vi "Motion Profile Generator-Target Speed-Demo.vi"(8 "Motion Profile Control Frame Rate":dbl=10.0, 9 "Target Speed":dbl=4.0, 10 "Max Jerk (rotations/sec^2)":dbl=1.0, 11 "Max Acceleration (rotations/sec)":dbl=3.0) -> (0 "XY Graph":cluster{dbl[], dbl[]}[](graph), 1 "jerk rotations/sec^3":dbl[](array[numeric]), 2 "acceleration rotations/sec^2":dbl[](array[numeric]), 3 "velocity rotations/sec":dbl[](array[numeric]))   [LabVIEW 2015]
panel:
  out "Final Speed":dbl
  # "This is just a trapezoidal motion profile generator"
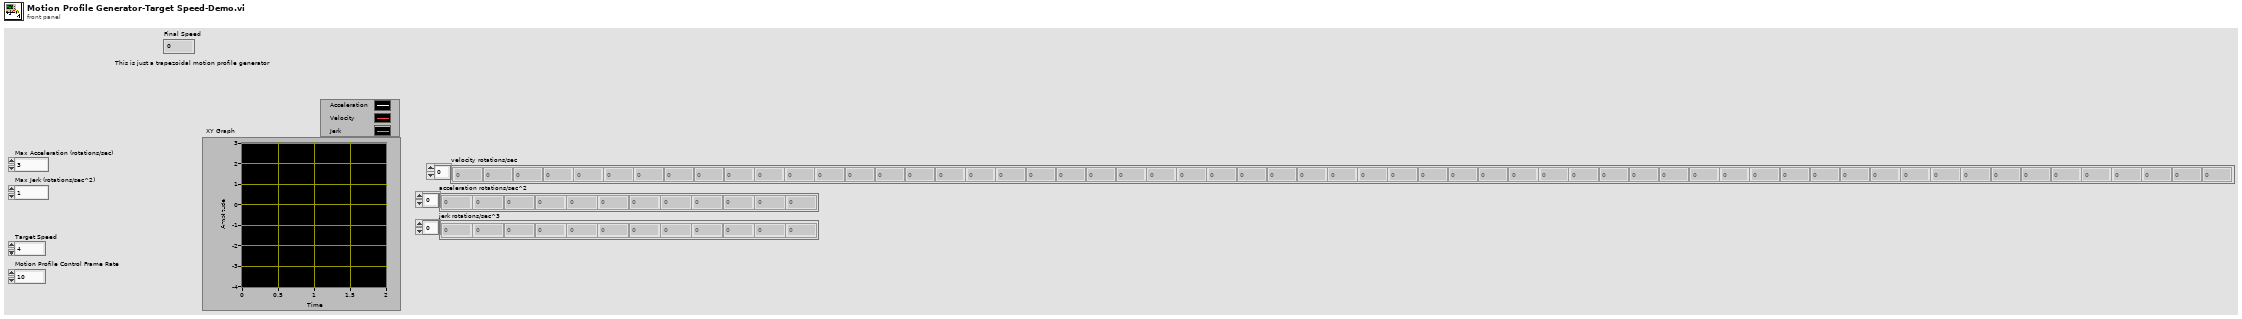
[diagram p1: front panel]
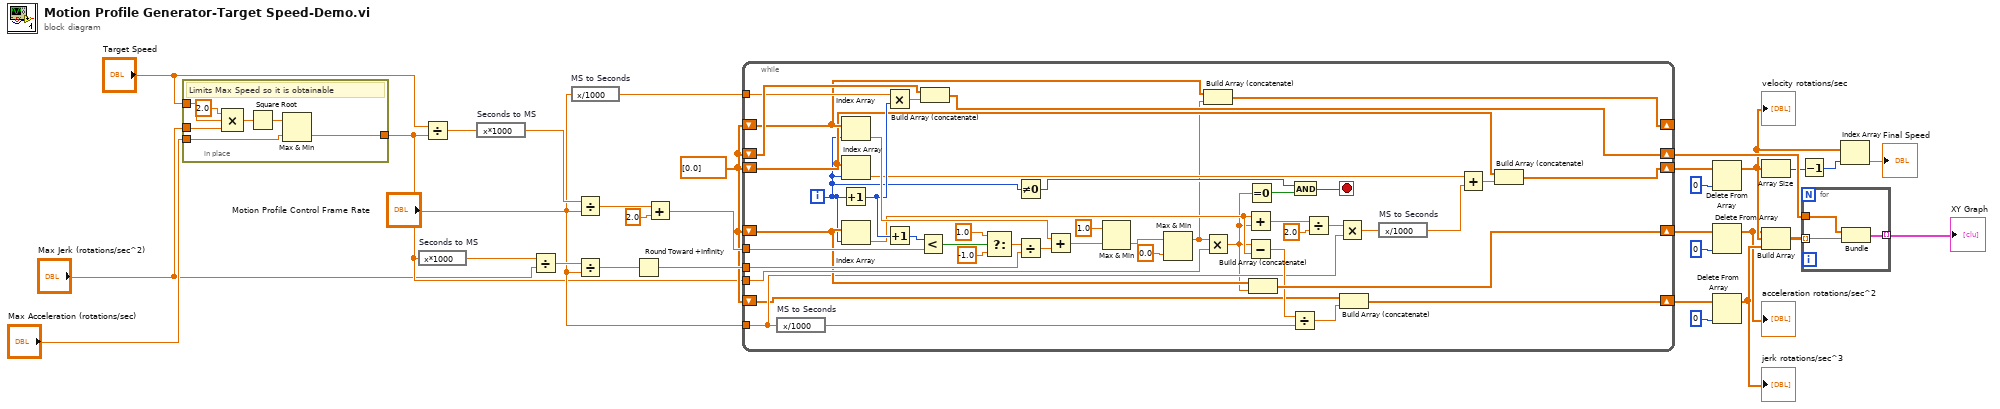
[diagram p0: block diagram]
diagram:
  w20 = dbl[] [0.0]
  n1 = in-place {
    in-place-border: "Max Acceleration (rotations/sec)" -> [w38]
    in-place-border: [w36] -> w12
    in-place-border: "Max Jerk (rotations/sec^2)" -> [w32]
    in-place-border: "Target Speed" -> [w33]
    # "Limits Max Speed so it is obtainable"
    n2 = Compound Arithmetic op=MULTIPLY(2.0 ("x"), w33, w32) -> (w35:dbl)
    n3 = Square Root(x=w35) -> (sqrt(x)=w34:dbl)
    n4 = Max & Min(x=w34, y=w38) -> (min(x,y)=w36:dbl)  [unwired: 1 out]
  }
  n5 = expression code="x*1000" "Seconds to MS"(w12) -> (w30:dbl)
  n6 = Divide(x="Target Speed", y=w12) -> (x/y=w29:dbl)
  n7 = expression code="x*1000" "Seconds to MS"(w29) -> (w28:dbl)
  n8 = Divide(x=w30, y="Max Jerk (rotations/sec^2)") -> (x/y=w24:dbl)
  n9 = expression code="x/1000" "MS to Seconds"("Motion Profile Control Frame Rate") -> (w31:dbl)
  n10 = Divide(x=w28, y="Motion Profile Control Frame Rate") -> (x/y=w27:dbl)
  n11 = Divide(x=w24, y="Motion Profile Control Frame Rate") -> (x/y=w23:dbl)
  n12 = Round Toward +Infinity(x=w23) -> (ceil(x): smallest int >= x=w22:dbl)
  n13 = Add(x=w27, y=2.0) -> (x+y=w25:dbl)
  n14 = while {
    shift-right: [w82] -> w18
    shift-left: w20 -> [w83]
    tunnel: w31 -> [w81]
    tunnel: w25 -> [w79]
    shift-right: [w65] -> _
    shift-left: w20 -> [w64]
    tunnel: w22 -> [w71]
    tunnel: w12 -> [w63]
    shift-right: [w62] -> w6
    shift-left: w20 -> [w60]
    shift-right: [w61] -> w4
    shift-left: w20 -> [w54]
    tunnel: "Motion Profile Control Frame Rate" -> [w48]
    shift-right: [w46] -> w8
    shift-left: w20 -> [w45]
    i -> [w44]
    stop <- w40 stop-if-true
    n15 = expression code="x/1000" "MS to Seconds"(w48) -> (w49:dbl)
    n16 = Index Array(array=w64, index=w44) -> (element=w69:dbl)
    n17 = Index Array(array=w54, index=w44) -> (element=w53:dbl)
    n18 = Increment(x=w44) -> (x+1=w67:i32)
    n19 = Index Array(array=w60, index=w44) -> (element=w51:dbl)
    n20 = Multiply(x=w81, y=w67) -> (x*y=w80:dbl)
    n21 = Increment(x=w67) -> (x+1=w68:i32)
    n22 = Less?(x=w68, y=w79) -> (x < y?=w75:bool)
    n23 = Build Array (concatenate)(w83, w80) -> (w82:dbl[])
    n24 = Select(t=1.0, s=w75, f=-1.0) -> (s? t:f=w72:dbl)
    n25 = Not Equal To 0?(x=w44) -> (x != 0?=w41:bool)
    n26 = Divide(x=w72, y=w71) -> (x/y=w70:dbl)
    n27 = Add(x=w69, y=w70) -> (x+y=w66:dbl)
    n28 = Max & Min(x=1.0, y=w66) -> (min(x,y)=w77:dbl)  [unwired: 1 out]
    n29 = Max & Min(x=w77, y=0.0) -> (max(x,y)=w39:dbl)  [unwired: 1 out]
    n30 = Build Array (concatenate)(w64, w39) -> (w65:dbl[])
    n31 = Multiply(x=w39, y=w63) -> (x*y=w43:dbl)
    n32 = Add(x=w51, y=w43) -> (x+y=w59:dbl)
    n33 = Subtract(x=w43, y=w51) -> (x-y=w50:dbl)
    n34 = Equal To 0?(x=w43) -> (x = 0?=w42:bool)
    n35 = Build Array (concatenate)(w60, w43) -> (w62:dbl[])
    n36 = Divide(x=w50, y=w49) -> (x/y=w47:dbl)
    n37 = And(x=w41, y=w42) -> (x .and. y?=w40:bool)
    n38 = Divide(x=w59, y=2.0) -> (x/y=w57:dbl)
    n39 = Multiply(x=w57, y=w48) -> (x*y=w56:dbl)
    n40 = Build Array (concatenate)(w45, w47) -> (w46:dbl[])
    n41 = expression code="x/1000" "MS to Seconds"(w56) -> (w55:dbl)
    n42 = Add(x=w53, y=w55) -> (x+y=w52:dbl)
    n43 = Build Array (concatenate)(w54, w52) -> (w61:dbl[])
  }
  n44 = Delete From Array(array=w4, index=0) -> (array with subset deleted=w3:dbl[])  [unwired: 1 in, 1 out]
  "velocity rotations/sec" <- w3
  n45 = Delete From Array(array=w6, index=0) -> (array with subset deleted=w2:dbl[])  [unwired: 1 in, 1 out]
  "acceleration rotations/sec^2" <- w2
  n46 = Delete From Array(array=w8, index=0) -> (array with subset deleted=w7:dbl[])  [unwired: 1 in, 1 out]
  "jerk rotations/sec^3" <- w7
  n47 = Array Size(array=w3) -> (size(s)=w16:i32)
  n48 = Build Array(w2, w3, w7) -> (w19:dbl[][])
  n49 = Decrement(x=w16) -> (x-1=w15:i32)
  n50 = for {
    tunnel: w19 -> [w86] mode=indexing
    tunnel: w18 -> [w85]
    tunnel: [w84] -> w17 mode=indexing
    n51 = Bundle(w85, w86) -> (w84:cluster{dbl[], dbl[]})  [unwired: 1 in]
  }
  "XY Graph" <- w17
  n52 = Index Array(array=w3, index=w15) -> (element=→"Final Speed":dbl)
